vi "Generate Channels.vi"(8 "error in (no error)":errorcluster, 11 "Lakeshore 218 in":refnum<class "Lakeshore 218.lvclass">) -> (0 "error out":errorcluster, 1 "Channel Names":string[](array[string])=["Telescope RA", "Telescope DEC", "Telescope Moving?", "Telescope Status"], 2 "Channel List":refnum<class "HK Item.lvclass">[](array[class]), 3 "Lakeshore 218 out":refnum<class "Lakeshore 218.lvclass">)   [LabVIEW 2022 SP3, in "Lakeshore 218.lvclass"]
uses:
  Lakeshore 218.lvclass
  hk-channel-class/hk-channel-class/HK Item/HK Item.lvclass
  Lakeshore 218.lvclass/Lakeshore 218.ctl
  hk-channel-class/hk-channel-class/HK Item/HK Channel Units and Setup.ctl
  hk-channel-class/hk-channel-class/HK Item/HK Channel enum Data Type.ctl
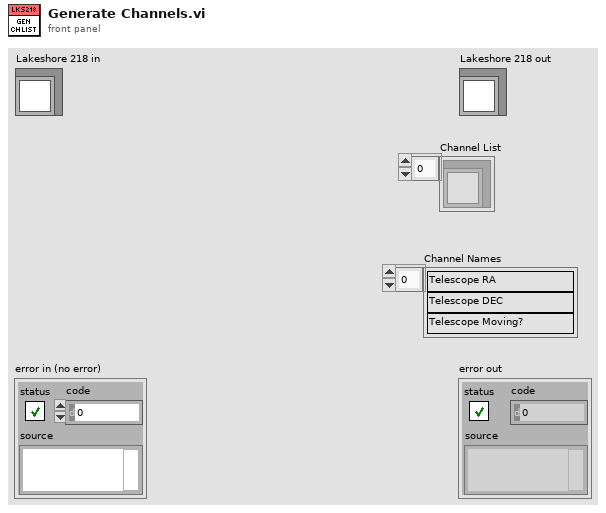
[diagram p1: front panel]
types:
  T1 = typedef "HK Item.lvclass/HK Channel Units and Setup.ctl" = cluster{"Unit Type":string, "Units":string, "Configuration":string, "Digits":i32, "Data Type":T2, "Exponential?":bool, "Source":string}
  T2 = typedef "HK Item.lvclass/HK Channel enum Data Type.ctl" = enum16{"Floating Point", "Integer", "Enum", "String", "Waveform", "File"}
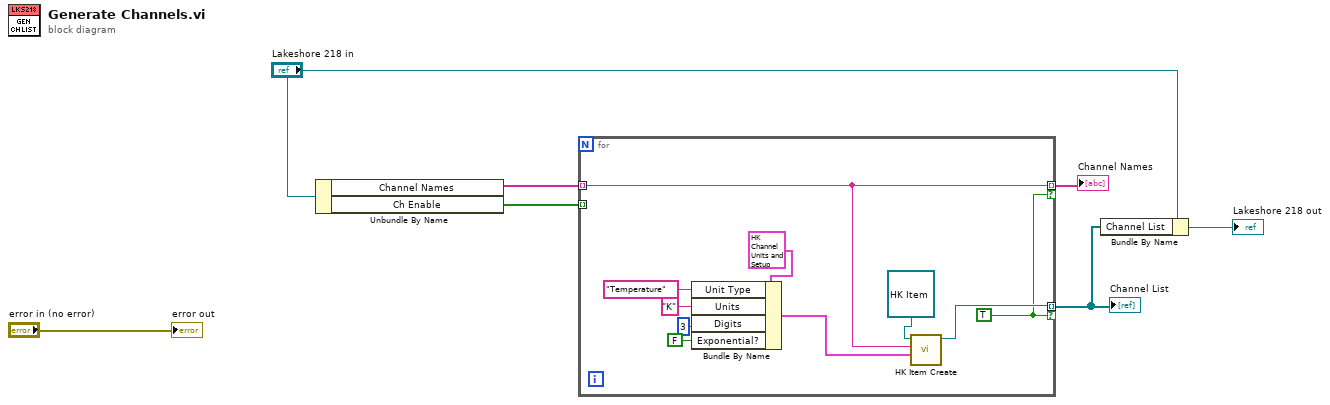
[diagram p0: block diagram]
diagram:
  n1 = Unbundle By Name("Lakeshore 218 in") -> ("Channel Names"=w6:string[], "Ch Enable"=w1:bool[])
  n2 = for {
    tunnel: w6 -> [w8] mode=indexing
    tunnel: [w16] -> w3 mode=indexing if=w15
    tunnel: [w8] -> w7 mode=indexing if=w15
    tunnel: w1 -> [_] mode=indexing
    w15 = TRUE
    n3 = Bundle By Name(cluster=T1 {"Unit Type"="", "Units"="", "Configuration"="", "Digits"=3, "Data Type"=enum."Floating Point", "Exponential?"=FALSE, "Source"=""} ("Channel Setup"), "Unit Type"="Temperature", "Units"="K", "Digits"=3, "Exponential?"=FALSE) -> (w9:T1)
    n4 = call-dynamic "HK Item Create.vi"("Channel Setup"=w9, "Name"=w8, "HK Item in"=refnum<class "HK Item.lvclass"> refnum) -> ("HK Item out"=w16:refnum<class "HK Item.lvclass">)  [unwired: 7 in, 1 out]
  }
  "Channel List" <- w3
  "Channel Names" <- w7
  n5 = Bundle By Name(cluster="Lakeshore 218 in", "Channel List"=w3) -> (→"Lakeshore 218 out":refnum<class "Lakeshore 218.lvclass">)
  "error out" <- "error in (no error)"
